vi "Cal Sets Catalog.vi"(8 "error in (no error)":errorcluster {"code" format="%.0x"}, 11 "instrument handle":refnum<k15>) -> (0 "error out":errorcluster {"code" format="%.0x"}, 2 "Val":string, 3 "instrument handle out":refnum<k15>)   [LabVIEW 2014, in "Agilent NA.lvlib"]
doc: "Returns a comma-separated the names of Cal Sets stored on the PNA."
uses:
  Agilent NA.lvlib
  AgNA.dll
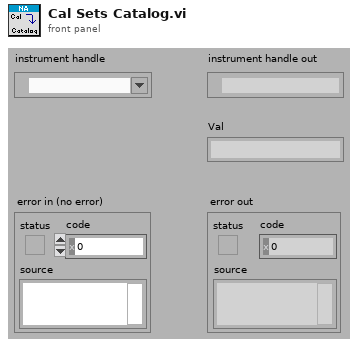
[diagram p1: front panel]
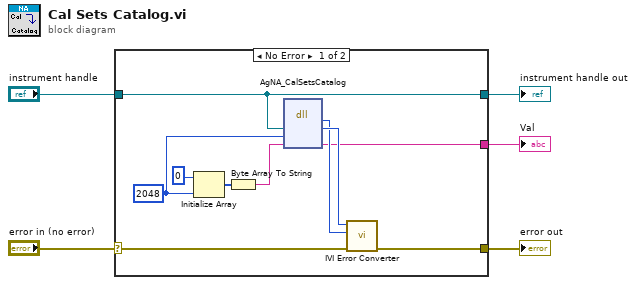
[diagram p0: block diagram]
diagram:
  n1 = case shown="No Error" "error in (no error)" {
    selector: "error in (no error)" -> [w13 w17]
    tunnel: [w12 w17] -> w5
    tunnel: [w8 _] -> w3
    tunnel: [w7 w16] -> w1
    tunnel: "instrument handle" -> [w7 w16]
    frame No Error {
      w6 = 2048 ("dimension size")
      n2 = Initialize Array(u8 0 ("element"), w6) -> (w10:u8[])
      n3 = Byte Array To String(unsigned byte array=w10) -> (string=w11:string)
      n4 = dll-call lib="AgNA**.dll" fn="AgNA_CalSetsCatalog"("Vi"=w7, "ValBufferSize"=w6, "Val"=w11) -> (w14:i32, "Vi"=w15:u32, "Val"=w8:string)  [unwired: 4 in, 2 out]
      n5 = call "IVI Error Converter.vi"("error in (no error)"=w13, "IVI error code (0)"=w14, "instrument handle"=w15) -> ("error out"=w12:errorcluster)  [unwired: 7 in, 1 out]
    }
    frame Error {
    }
  }
  "error out" <- w5
  "instrument handle out" <- w1
  "Val" <- w3
